vi "Calculate BER.vi"(0 "error count":u64, 5 "sample count":u64) -> (4 "BER":dbl)   [LabVIEW 2015, in "niHighSpeedSerial Eye Scan Common v1 Host.lvlib"]
uses:
  <instrlib>/niHighSpeedSerial/Eye Scan/v1/Host/Common/niHighSpeedSerial Eye Scan Common v1 Host.lvlib
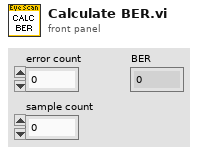
[diagram p1: front panel]
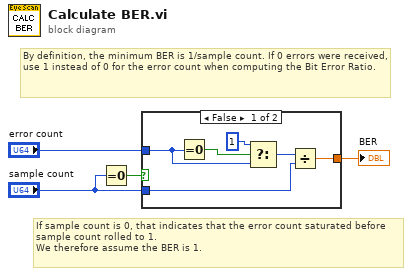
[diagram p0: block diagram]
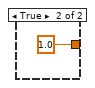
[diagram p2: hidden frame]
diagram:
  # "If sample count is 0, that indicates that the error count saturated before sample count rolled to 1.\nWe therefore assume the BER is 1."
  # "By definition, the minimum BER is 1/sample count. If 0 errors were received, use 1 instead of 0 for the error count when computing the Bit Error Ratio."
  n1 = Equal To 0?(x="sample count") -> (x = 0?=w2:bool)
  n2 = case shown="False" w2 {
    tunnel: [w9 1.0 ("t")] -> w4
    tunnel: "sample count" -> [w10 _]
    tunnel: "error count" -> [w5 _]
    frame False {
      n3 = Equal To 0?(x=w5) -> (x = 0?=w8:bool)
      n4 = Select(t=u64 1 ("f"), s=w8, f=w5) -> (s? t:f=w6:u64)
      n5 = Divide(x=w6, y=w10) -> (x/y=w9:dbl)
    }
    frame True {
    }
  }
  "BER" <- w4
